vi "initialize ASI stage.vi"(5 "y range":dbl, 6 "z range":dbl, 7 "x range":dbl, 8 "error in (no error)":errorcluster, 9 "timeout":u32=100, 10 "Baud rate":u32=115200, 11 "VISA resource name":refnum<visa-resource-name>) -> (0 "error out":errorcluster, 3 "ASI stage":T1)   [LabVIEW 2010]
uses:
  stage properties.ctl
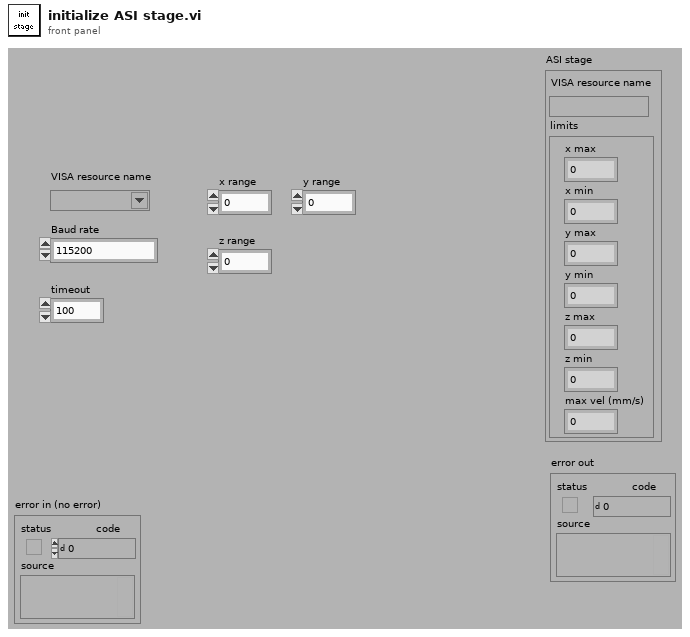
[diagram p1: front panel]
types:
  T1 = typedef "stage properties.ctl" = cluster{"VISA resource name":refnum<visa-resource-name>, "limits":cluster{"x max":dbl, "x min":dbl, "y max":dbl, "y min":dbl, "z max":dbl, "z min":dbl, "max vel (mm/s)":dbl}}
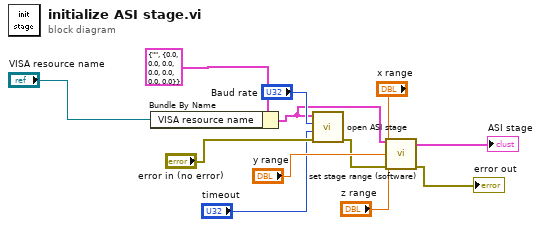
[diagram p0: block diagram]
diagram:
  n1 = Bundle By Name(cluster=T1 {"VISA resource name"="", "limits"={"x max"=0.0, "x min"=0.0, "y max"=0.0, "y min"=0.0, "z max"=0.0, "z min"=0.0, "max vel (mm/s)"=0.0}} ("ASI stage"), "VISA resource name"="VISA resource name") -> (w2:T1)
  n2 = call "open ASI stage.vi"("error in (no error)"="error in (no error)", "timeout"="timeout", "Baud rate"="Baud rate", "ASI stage"=w2) -> ("error out"=w3:errorcluster)  [unwired: 7 in]
  n3 = call "set stage range (software).vi"("ASI stage"=w2, "x range"="x range", "y range"="y range", "z range"="z range", "error in (no error)"=w3) -> ("ASI stage out"=→"ASI stage":T1, "error out"=→"error out":errorcluster)  [unwired: 9 in]
